vi "Execute Control Visible Toggle.vi"(6 "Mouse Position":T1 caption="鼠标位置", 8 "User VI Ref":refnum<vi> caption="用户VI引用", 9 "Menu Item Tag Suffix":string caption="菜单项标签后缀", 10 "Remaining Items":refnum<vi>[](array[refnum]) caption="剩余项", 11 "Affected Items":T2 caption="受影响的项") -> (0 "Fail transaction?":bool caption="操作失败？")   [LabVIEW 2020]
doc: "该VI属于修改LabVIEW快捷菜单部分。这是用户选择快捷菜单时调用的执行VI。该VI执行选中菜单项的操作。"
uses:
  Control Visible Toggle.ctl
  <vilib>/Utility/miscctls.llb/LVPositionTypeDef.ctl
panel:
  # "除“受影响的项”之外，前面板上的其他所有控件都已锁定，以防被意外编辑。修改控件名称或类型，而不是“受影响的项”簇的元素将使VI无法作为菜单插件使用。\n\n请参考每个控件的即时帮助了解其用法。"
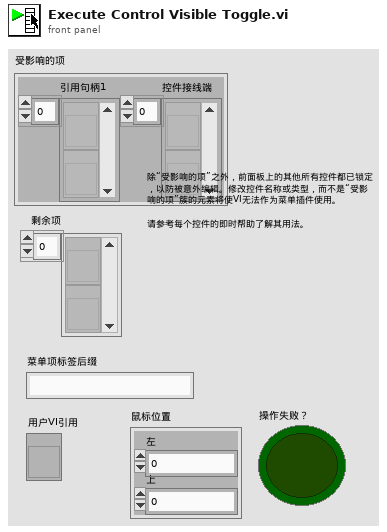
[diagram p1: front panel]
types:
  T1 = typedef "LVPositionTypeDef.ctl" = cluster{"Left":i32, "Top":i32}
  T2 = typedef "Control Visible Toggle.ctl" = cluster{"Control":refnum<vi>[], "Control Term":refnum<vi>[]}
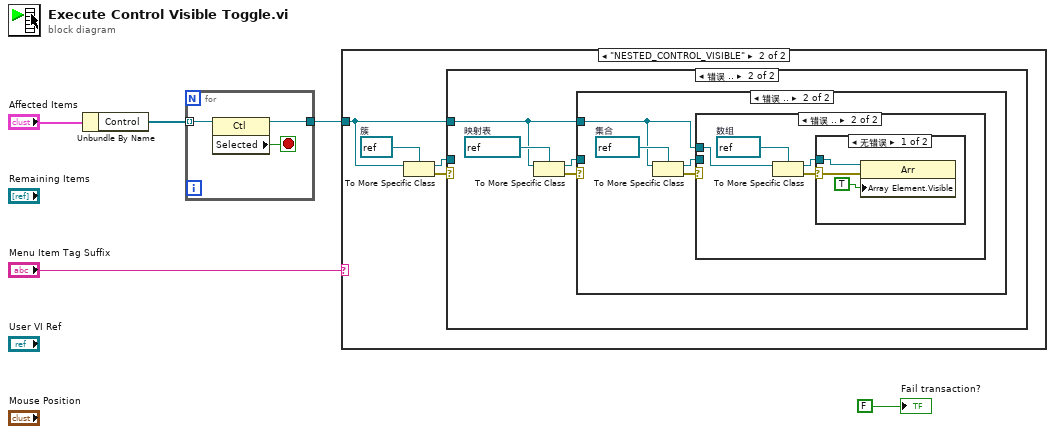
[diagram p0: block diagram]
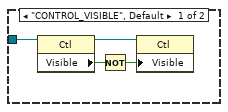
[diagram p2: hidden frame]
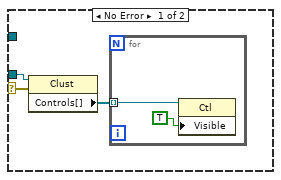
[diagram p3: hidden frame]
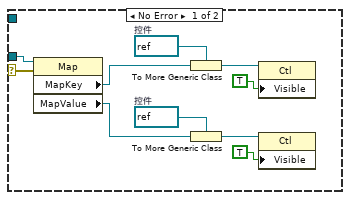
[diagram p4: hidden frame]
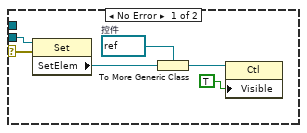
[diagram p5: hidden frame]
diagram:
  n1 = Unbundle By Name("Affected Items") -> ("Control"=w3:refnum<vi>[])
  n2 = for {
    tunnel: w3 -> [w8] mode=indexing
    tunnel: [w7] -> w2
    stop <- w6 stop-if-true
    n3 = property class="Ctl"(reference=w8) -> (reference out=w7:refnum<vi>, "Selected"=w6:bool)  [unwired: 1 in, 1 out]
  }
  n4 = case shown="\"NESTED_CONTROL_VISIBLE\"" "Menu Item Tag Suffix" {
    tunnel: w2 -> [w9 w13]
    frame "CONTROL_VISIBLE", Default {
      n5 = property class="Ctl"(reference=w9) -> (reference out=w12:refnum<vi>, "Visible"=w11:bool)  [unwired: 1 in, 1 out]
      n6 = Not(x=w11) -> (.not. x?=w10:bool)
      n7 = property class="Ctl"(reference=w12, "Visible"=w10) -> ()  [unwired: 1 in, 2 out]
    }
    frame "NESTED_CONTROL_VISIBLE" {
      w16 = refnum<vi> refnum  # 簇
      n8 = To More Specific Class(target class=w16, reference=w13) -> (specific class reference=w14:refnum<vi>, error out=w15:errorcluster)  [unwired: 1 in]
      n9 = case shown="错误 .." w15 {
        selector: w15 -> [w17 _]
        tunnel: w13 -> [_ w24]
        tunnel: w14 -> [w19 _]
        frame No Error {
          n10 = property class="Clust"(reference=w19, error in=w17) -> ("Controls[]"=w18:refnum<vi>[])  [unwired: 2 out]
          n11 = for {
            tunnel: w18 -> [w21] mode=indexing
            n12 = property class="Ctl"(reference=w21, "Visible"=TRUE ("可见")) -> ()  [unwired: 1 in, 2 out]
          }
        }
        frame Error {
          w25 = refnum<vi> refnum  # 映射表
          n13 = To More Specific Class(target class=w25, reference=w24) -> (specific class reference=w22:refnum<vi>, error out=w23:errorcluster)  [unwired: 1 in]
          n14 = case shown="错误 .." w23 {
            selector: w23 -> [w35 _]
            tunnel: w24 -> [_ w38]
            tunnel: w22 -> [w34 _]
            frame No Error {
              w27 = refnum<vi> refnum  # 控件
              w33 = refnum<vi> refnum  # 控件
              n15 = property class="Map"(reference=w34, error in=w35) -> ("MapKey"=w30:refnum<vi>, "MapValue"=w26:refnum<vi>)  [unwired: 2 out]
              n16 = To More Generic Class(target class=w33, reference=w30) -> (generic class reference=w32:refnum<vi>)
              n17 = To More Generic Class(target class=w27, reference=w26) -> (generic class reference=w28:refnum<vi>)
              n18 = property class="Ctl"(reference=w32, "Visible"=TRUE ("可见")) -> ()  [unwired: 1 in, 2 out]
              n19 = property class="Ctl"(reference=w28, "Visible"=TRUE ("可见")) -> ()  [unwired: 1 in, 2 out]
            }
            frame Error {
              w39 = refnum<vi> refnum  # 集合
              n20 = To More Specific Class(target class=w39, reference=w38) -> (specific class reference=w36:refnum<vi>, error out=w37:errorcluster)  [unwired: 1 in]
              n21 = case shown="错误 .." w37 {
                selector: w37 -> [w44 _]
                tunnel: w38 -> [_ w47]
                tunnel: w36 -> [w45 _]
                frame No Error {
                  w43 = refnum<vi> refnum  # 控件
                  n22 = property class="Set"(reference=w45, error in=w44) -> ("SetElem"=w40:refnum<vi>)  [unwired: 2 out]
                  n23 = To More Generic Class(target class=w43, reference=w40) -> (generic class reference=w42:refnum<vi>)
                  n24 = property class="Ctl"(reference=w42, "Visible"=TRUE ("可见")) -> ()  [unwired: 1 in, 2 out]
                }
                frame Error {
                  w49 = refnum<vi> refnum  # 数组
                  n25 = To More Specific Class(target class=w49, reference=w47) -> (specific class reference=w46:refnum<vi>, error out=w48:errorcluster)  [unwired: 1 in]
                  n26 = case shown="无错误" w48 {
                    selector: w48 -> [w50 _]
                    tunnel: w46 -> [w52 _]
                    frame No Error {
                      n27 = property class="Arr"(reference=w52, error in=w50, "Array Element.Visible"=TRUE ("数组元素.可见")) -> ()  [unwired: 2 out]
                    }
                    frame Error {
                    }
                  }
                }
              }
            }
          }
        }
      }
    }
  }
  "Fail transaction?" <- FALSE ("Fail transaction?")
